vi "Read State.vi"(8 "error in (no error)":errorcluster, 11 "Expansion in":refnum<class "Saturation.lvclass">) -> (0 "error out":errorcluster, 2 "State":T1, 3 "Expansion out":refnum<class "Saturation.lvclass">)   [LabVIEW 2017, in "Saturation.lvclass"]
uses:
  Saturation.lvclass
  Type Defs/Saturation State.ctl
  Saturation.lvclass/Saturation.ctl
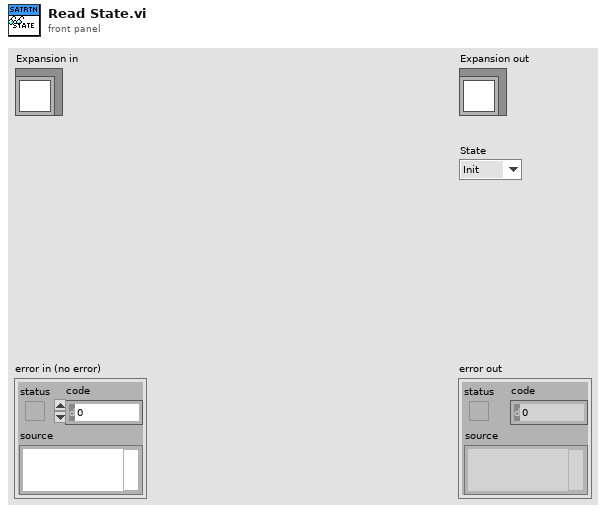
[diagram p1: front panel]
types:
  T1 = typedef "Saturation.lvclass/Saturation State.ctl" = enum16{"Init", "Update", "Go", "Control Valve", "Wait for Pressure", "Wait and Monitor", "Stop", "Idle", "Error", "Shutdown"}
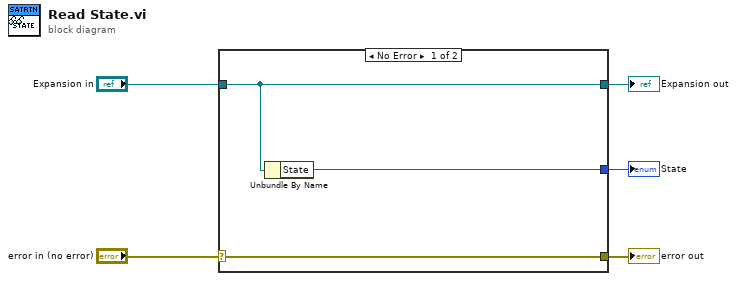
[diagram p0: block diagram]
diagram:
  n1 = case shown="No Error" "error in (no error)" {
    selector: "error in (no error)" -> [w8 w9]
    tunnel: [w8 w9] -> w4
    tunnel: [w7 w10] -> w2
    tunnel: "Expansion in" -> [w7 w10]
    tunnel: [w6 _] -> w1
    frame No Error {
      n2 = Unbundle By Name(w7) -> ("State"=w6:T1)
    }
    frame Error {
    }
  }
  "error out" <- w4
  "Expansion out" <- w2
  "State" <- w1
